vi "TDK工况电流.vi"() -> ()   [LabVIEW 2021]
uses:
  <instrlib>/Keithley 27XX/Public/Data/Read Single Point.vi
  <instrlib>/TDK-Lambda G Series/TDK-Lambda G Series.lvlib
  <vilib>/Utility/file.llb/Read Delimited Spreadsheet (DBL).vi
  <instrlib>/Keithley 27XX/Keithley 27XX.lvlib
panel:
  in  "时间":dbl=20.0 caption="延迟时间(s)"
  in  "电流":dbl
  out "all rows":dbl[][](array[numeric]) caption="加载电流"
  out "实际电流":dbl[](array[numeric]) format="%#.6g"
  in  "2700":refnum<visa-resource-name>="GPIB0::16::INSTR"
  in  "TDK地址":refnum<visa-resource-name>="COM15"
  in  "file path (dialog if empty)":path caption="电流加载"
  in  "电源台数":dbl=3.0
  in  "循环次数":i32=1
  in  "?":bool
  out "已完成循环次数":i32
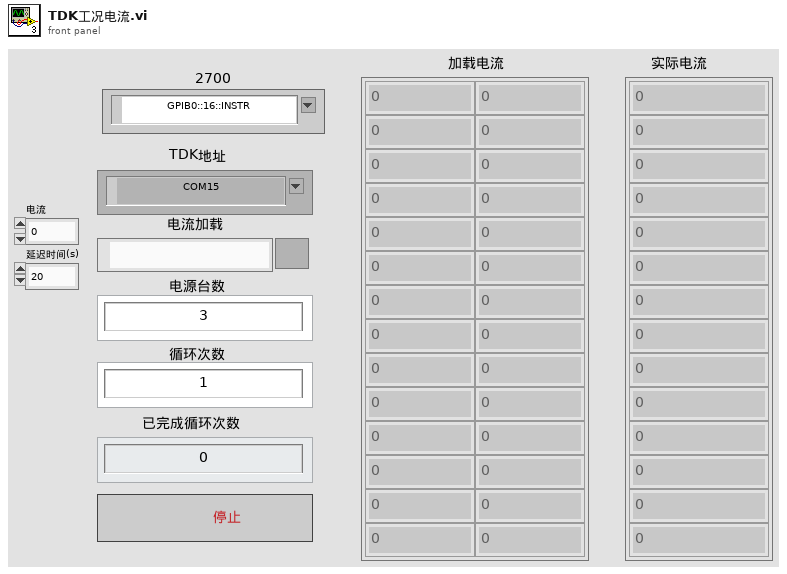
[diagram p1: front panel]
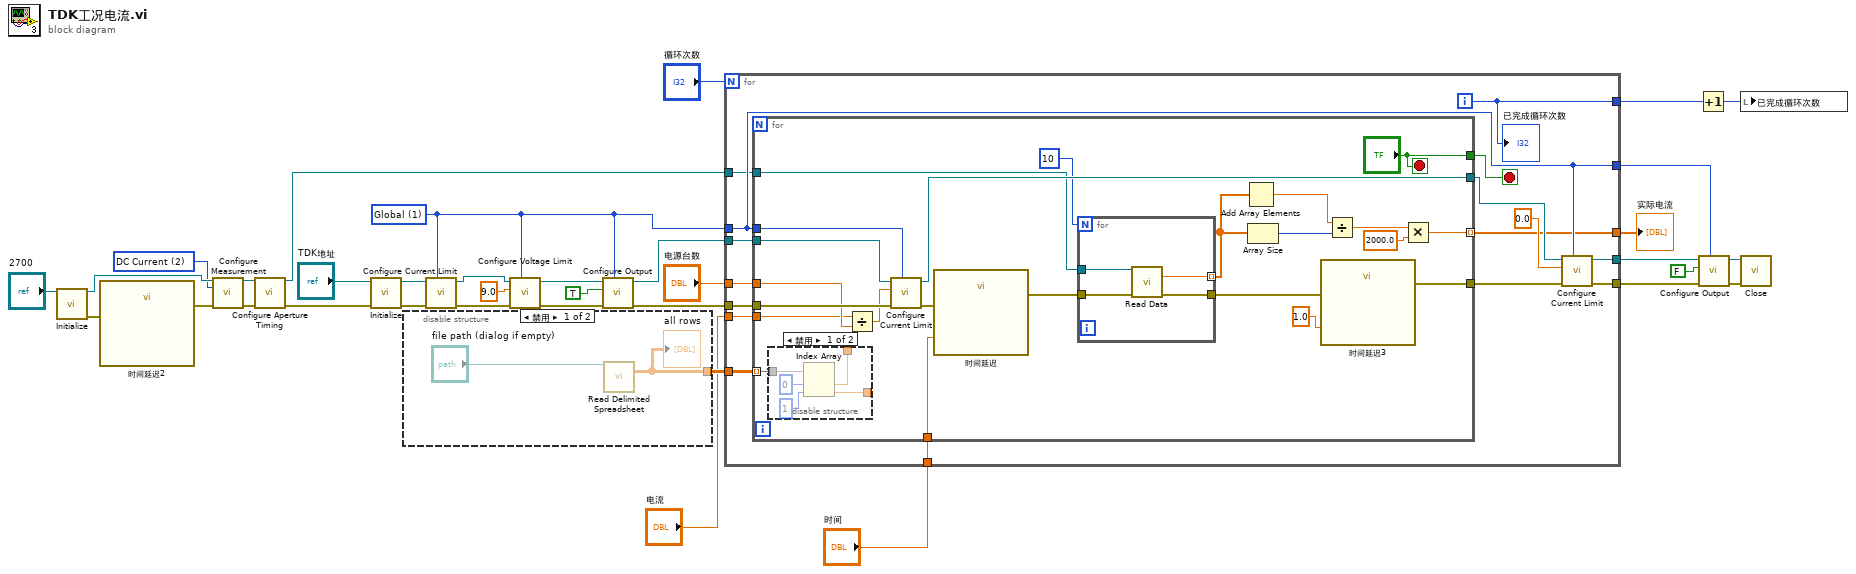
[diagram p0: block diagram]
diagram:
  w8 = u16 2 items=["DC Voltage", "AC Voltage", "DC Current", "AC Current", "Resistance", "Four-Wire Resistance", "Temperature", "Frequency", "Period", "Continuity"] ("Function (0: DC Voltage)")
  w18 = u16 1 items=["Single", "Global"] ("Globalize (0: Single)")
  n1 = call <instrlib>:"Initialize.vi"("VISA resource name"="2700") -> ("VISA resource name out"=w10:refnum<visa-resource-name>, "error out"=w11:errorcluster)  [unwired: 13 in]
  n2 = call "时间延迟2"("error in (no error)"=w11) -> ("error out"=w9:errorcluster)  [unwired: 10 in]
  n3 = call <instrlib>:"Configure Measurement.vi"("VISA resource name"=w10, "Function (0: DC Voltage)"=w8, "error in (no error)"=w9) -> ("VISA resource name out"=w7:refnum<visa-resource-name>, "error out"=w6:errorcluster)  [unwired: 11 in]
  n4 = call <instrlib>:"Configure Aperture Timing.vi"("VISA resource name"=w7, "error in (no error)"=w6) -> ("VISA resource name out"=w4:refnum<visa-resource-name>, "error out"=w5:errorcluster)  [unwired: 12 in]
  n5 = call <instrlib>:"Initialize.vi"("error in (no error)"=w5, "VISA resource name"="TDK地址") -> ("error out"=w32:errorcluster, "VISA resource name out"=w33:refnum<visa-resource-name>)  [unwired: 8 in]
  n6 = disable-structure shown="禁用" {
    disable-tunnel: [w36 _] -> w13
    frame Disabled {
      n7 = call-poly <vilib>:"Read Delimited Spreadsheet.vi"("file path (dialog if empty)"="file path (dialog if empty)") -> ("all rows"=w36:dbl[][])  [unwired: 9 in, 5 out]
      "all rows" <- w36
    }
    frame Enabled {
    }
  }
  n8 = call <instrlib>:"Configure Current Limit.vi"("Globalize (0: Single)"=w18, "error in (no error)"=w32, "VISA resource name"=w33) -> ("error out"=w31:errorcluster, "VISA resource name out"=w30:refnum<visa-resource-name>)  [unwired: 7 in]
  n9 = call <instrlib>:"Configure Voltage Limit.vi"("Globalize (0: Single)"=w18, "error in (no error)"=w31, "Voltage Limit (0V)"=9.0 ("Voltage Level (0.0 V)"), "VISA resource name"=w30) -> ("error out"=w25:errorcluster, "VISA resource name out"=w26:refnum<visa-resource-name>)  [unwired: 6 in]
  n10 = call <instrlib>:"Configure Output.vi"("Globalize (0: Single)"=w18, "error in (no error)"=w25, "Enable Output (False)"=TRUE, "VISA resource name"=w26) -> ("error out"=w22:errorcluster, "VISA resource name out"=w23:refnum<visa-resource-name>)  [unwired: 6 in]
  n11 = for {
    N: "循环次数" -> [_]
    tunnel: w13 -> [w46]
    tunnel: w18 -> [w45]
    tunnel: [w45] -> w17
    tunnel: [w44] -> w16
    tunnel: "电源台数" -> [w43]
    tunnel: w4 -> [w41]
    tunnel: w22 -> [w49]
    tunnel: [w48] -> w20
    tunnel: w23 -> [w51]
    tunnel: [w47] -> w21
    tunnel: [w40] -> w3
    tunnel: "电流" -> [w39]
    tunnel: "时间" -> [w38]
    i -> [w44]
    stop <- w42 stop-if-true
    n12 = for {
      tunnel: w46 -> [w76] mode=indexing
      tunnel: w51 -> [w75]
      tunnel: w49 -> [w74]
      tunnel: [w61] -> w53
      tunnel: [w72] -> w52
      tunnel: w45 -> [w71]
      tunnel: w43 -> [w69]
      tunnel: ["?"] -> w42
      tunnel: w41 -> [w67]
      tunnel: [w64] -> w40 mode=indexing
      tunnel: w39 -> [w55]
      tunnel: w38 -> [w54]
      stop <- "?" stop-if-true
      n13 = disable-structure shown="禁用" {
        disable-tunnel: w76 -> [w81 _]
        disable-tunnel: [w78 _] -> _
        disable-tunnel: [w77 _] -> _
        frame Disabled {
          n14 = Index Array(array=w81, index #1=0 ("索引"), index #2=1 ("索引")) -> (element #1=w77:dbl, element #2=w78:dbl)
        }
        frame Enabled {
        }
      }
      n15 = Divide(x=w55, y=w69) -> (x/y=w70:dbl)
      n16 = call <instrlib>:"Configure Current Limit.vi"("Globalize (0: Single)"=w71, "error in (no error)"=w74, "Current Limit (0A)"=w70, "VISA resource name"=w75) -> ("error out"=w73:errorcluster, "VISA resource name out"=w72:refnum<visa-resource-name>)  [unwired: 6 in]
      n17 = call "时间延迟"("error in (no error)"=w73, "Delay Time (s)"=w54) -> ("error out"=w66:errorcluster)  [unwired: 9 in]
      n18 = for {
        N: 10 -> [_]
        tunnel: w67 -> [w85]
        tunnel: [w83] -> w58 mode=indexing
        tunnel: w66 -> [w84]
        tunnel: [w82] -> w62
        n19 = call-poly <instrlib>:"Read Data.vi"("VISA resource name"=w85, "error in (no error)"=w84) -> ("Measurement Data"=w83:dbl, "error out"=w82:errorcluster)  [unwired: 11 in, 1 out]
      }
      n20 = Add Array Elements(numeric array=w58) -> (sum=w59:dbl)
      n21 = Array Size(array=w58) -> (size(s)=w57:i32)
      n22 = call "时间延迟3"("error in (no error)"=w62, "Delay Time (s)"=1.0) -> ("error out"=w61:errorcluster)  [unwired: 9 in]
      n23 = Divide(x=w59, y=w57) -> (x/y=w56:dbl)
      n24 = Multiply(x=w56, y=2000.0) -> (x*y=w64:dbl)
    }
    n25 = call <instrlib>:"Configure Current Limit.vi"("Globalize (0: Single)"=w45, "error in (no error)"=w53, "Current Limit (0A)"=0.0, "VISA resource name"=w52) -> ("error out"=w48:errorcluster, "VISA resource name out"=w47:refnum<visa-resource-name>)  [unwired: 6 in]
    "已完成循环次数" <- w44
  }
  "实际电流" <- w3
  n26 = Increment(x=w16) -> (x+1=w15:i32)
  n27 = call <instrlib>:"Configure Output.vi"("Globalize (0: Single)"=w17, "error in (no error)"=w20, "Enable Output (False)"=FALSE ("Enable Output (True)"), "VISA resource name"=w21) -> ("error out"=w27:errorcluster, "VISA resource name out"=w28:refnum<visa-resource-name>)  [unwired: 6 in]
  n28 = local write "已完成循环次数"(w15) -> ()
  n29 = call <instrlib>:"Close.vi"("error in (no error)"=w27, "VISA resource name"=w28) -> ()  [unwired: 9 in, 1 out]
